vi "dfd_Super Narrowband Filter Design Compute M and New Filter Type.vi"(7 "filter type":T2(ring), 9 "fc":dbl, 10 "fstop":dbl, 11 "fpass":dbl) -> (1 "M":i32, 3 "new filter type":T1(ring))   [LabVIEW 2017, in "NI_DigFilter_Process.lvlib"]
doc: "Gets the narrowband filter type for processing and multirate factor for design the super narrowband filter."
uses:
  <vilib>/addons/Digital Filter Design/NI_DigFilter_Process.lvlib
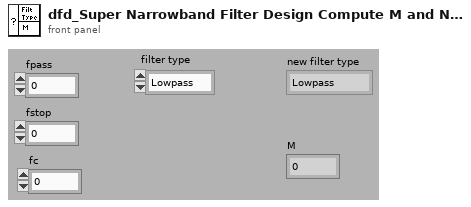
[diagram p1: front panel]
types:
  T1 = enum32{"Lowpass", "Highpass", "Bandpass", "Bandstop", "Wideband-Lowpass", "Wideband-Highpass"}
  T2 = enum16{"Lowpass", "Highpass", "Bandpass", "Bandstop"}
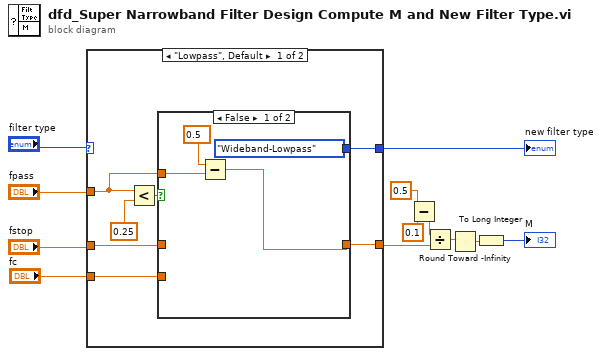
[diagram p0: block diagram]
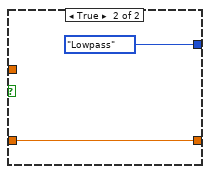
[diagram p2: hidden frame]
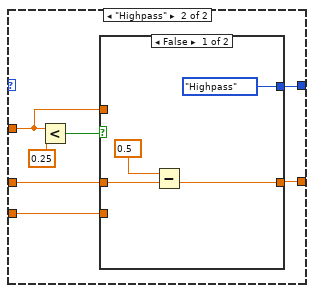
[diagram p3: hidden frame]
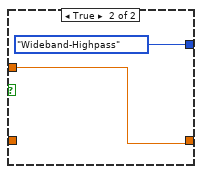
[diagram p4: hidden frame]
diagram:
  n1 = case shown="\"Lowpass\", Default" "filter type" {
    tunnel: "fpass" -> [w15 w29]
    tunnel: "fstop" -> [w14 w28]
    tunnel: [w17 w27] -> w4
    tunnel: [w16 w30] -> w5
    tunnel: "fc" -> [w13 w26]
    frame "Lowpass", Default {
      n2 = Less?(x=w15, y=0.25) -> (x < y?=w18:bool)
      n3 = case shown="False" w18 {
        tunnel: [T1."Wideband-Lowpass" ("filter type") T1."Lowpass" ("filter type")] -> w17
        tunnel: w14 -> [_ w24]
        tunnel: w15 -> [w21 _]
        tunnel: [w22 w24] -> w16
        tunnel: w13 -> [_ _]
        frame False {
          n4 = Subtract(x=0.5, y=w21) -> (x-y=w22:dbl)
        }
        frame True {
        }
      }
    }
    frame "Highpass" {
      n5 = Less?(x=w29, y=0.25) -> (x < y?=w31:bool)
      n6 = case shown="False" w31 {
        tunnel: w29 -> [_ w37]
        tunnel: w28 -> [w34 _]
        tunnel: [w35 w37] -> w30
        tunnel: [T1."Highpass" ("filter type") T1."Wideband-Highpass" ("filter type")] -> w27
        tunnel: w26 -> [_ _]
        frame False {
          n7 = Subtract(x=0.5, y=w34) -> (x-y=w35:dbl)
        }
        frame True {
        }
      }
    }
  }
  "new filter type" <- w4
  n8 = Subtract(x=0.5 ("y"), y=0.1) -> (x-y=w1:dbl)
  n9 = Divide(x=w1, y=w5) -> (x/y=w10:dbl)
  n10 = Round Toward -Infinity(1:w10) -> (0:w11:dbl)
  n11 = To Long Integer(number=w11) -> (32bit integer=→"M":i32)
